vi "题目8.vi"() -> ()   [LabVIEW 2017]
panel:
  in  "停止":bool
  out "单位 秒":dbl
  in  "字符串":string
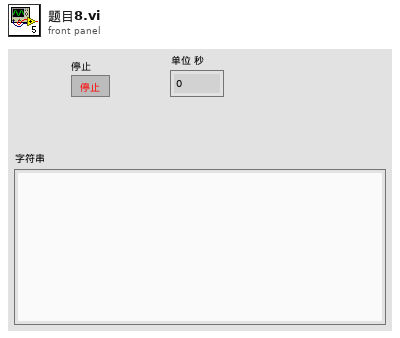
[diagram p1: front panel]
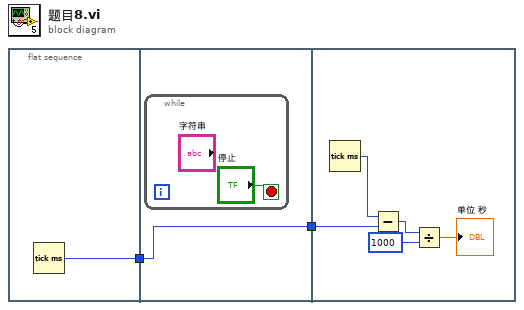
[diagram p0: block diagram]
diagram:
  n1 = flat-sequence {
    tunnel: [w3] -> w2
    tunnel: w2 -> [w4]
    tunnel: [w4] -> w1
    tunnel: w1 -> [w6]
    frame #0 {
      n2 = Tick Count (ms)() -> (millisecond timer value=w3:u32)
    }
    frame #1 {
      n3 = while {
        stop <- "停止" stop-if-true
      }
    }
    frame #2 {
      n4 = Tick Count (ms)() -> (millisecond timer value=w10:u32)
      n5 = Subtract(x=w10, y=w6) -> (x-y=w9:u32)
      n6 = Divide(x=w9, y=u32 1000) -> (x/y=→"单位 秒":dbl)
    }
  }
